vi "Create_AO_Signal4Z.vi"(8 "error in":errorcluster, 10 "AO Amplitude":dbl(slide) min=0.0 max=100.0 step=1.0 scale=0.0..100.0, 11 "ON / OFF":bool=TRUE) -> (0 "error out":errorcluster, 3 "WF":dbl[](array[numeric]))   [LabVIEW 2025]
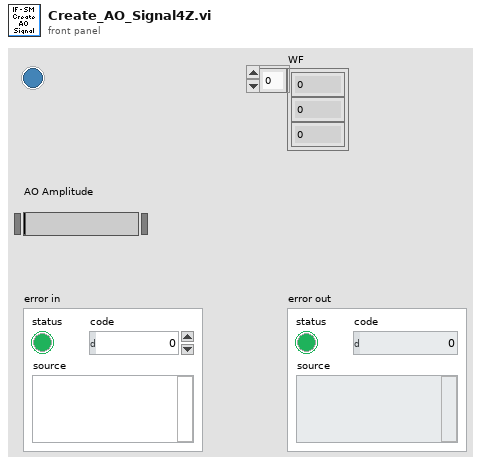
[diagram p1: front panel]
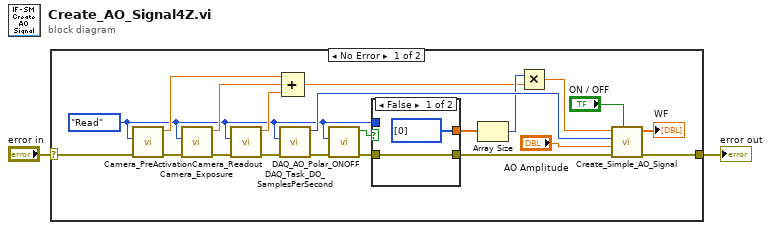
[diagram p0: block diagram]
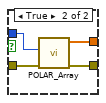
[diagram p2: hidden frame]
diagram:
  n1 = case shown="No Error" "error in" {
    selector: "error in" -> [w23 w30]
    tunnel: [w14 w30] -> w1
    frame No Error {
      w6 = enum16{"Init", "Write", "Read"}."Read" ("Action")
      n2 = call "Camera_PreActivation.vi"("error in"=w23, "Action"=w6) -> ("error out"=w22:errorcluster, "Camera_PreActivation"=w18:dbl)  [unwired: 8 in]
      n3 = call "Camera_Exposure.vi"("error in"=w22, "Action"=w6) -> ("error out"=w21:errorcluster, "Exposure (s)"=w17:dbl)  [unwired: 8 in]
      n4 = call "Camera_Readout.vi"("error in"=w21, "Action"=w6) -> ("error out"=w20:errorcluster, "Camera_Readout"=w12:dbl)  [unwired: 8 in]
      n5 = call "DAQ_Task_DO_SamplesPerSecond.vi"("error in"=w20, "Action"=w6) -> ("error out"=w5:errorcluster, "DO_Task_SamplesPerSec"=w15:u32)  [unwired: 8 in]
      n6 = Compound Arithmetic op=ADD(w18, w17, w12) -> (w9:dbl)
      n7 = call "DAQ_AO_Polar_ONOFF.vi"("error in"=w5, "Action"=w6) -> ("error out"=w4:errorcluster, "ON / OFF"=w7:bool)  [unwired: 8 in]
      n8 = case shown="False" w7 {
        tunnel: [u8[] [0] w29] -> w11
        tunnel: w6 -> [_ w28]
        tunnel: w4 -> [w25 w27]
        tunnel: [w25 w26] -> w3
        frame False {
        }
        frame True {
          n9 = call "POLAR_Array.vi"("error in"=w27, "Action"=w28) -> ("error out"=w26:errorcluster, "Pockels_Array"=w29:dbl[])  [unwired: 8 in]
        }
      }
      n10 = Array Size(array=w11) -> (size(s)=w10:i32)
      n11 = Multiply(x=w10, y=w9) -> (x*y=w8:dbl)
      n12 = call "Create_Simple_AO_Signal.vi"("On/OFF"="ON / OFF", "error in"=w3, "Amplitude"="AO Amplitude", "Samples / s (10000)"=w15, "Time (s)"=w8) -> ("error out"=w14:errorcluster, "Signal"=→"WF":dbl[])  [unwired: 5 in]
    }
    frame Error {
    }
  }
  "error out" <- w1
